vi "open SADI LV.vi"(10 "deviceNumber":i32, 11 "instance":i32) -> (3 "function return":u32)   [LabVIEW 2025, in "SADI_FW3.lvlib"]
doc: "SADI_API_Wrapper FT_STATUS openSADI_LV(int instance,int deviceNumber);"
uses:
  SADI_FW3.lvlib
  SADI_FW3.dll
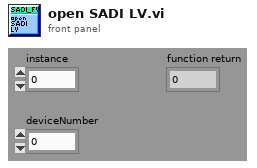
[diagram p1: front panel]
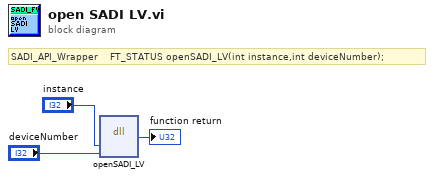
[diagram p0: block diagram]
diagram:
  # "SADI_API_Wrapper    FT_STATUS openSADI_LV(int instance,int deviceNumber);"
  n1 = dll-call lib="C:/Users/noaht/iCloudDrive/#1 School/Fall 2025/Controls Lab/LabView/EML4314c_FA25_framework_0/LVLib/SADI_FW3.*" fn="openSADI_LV"("instance"="instance", "deviceNumber"="deviceNumber") -> (→"function return":u32)  [unwired: 5 in, 2 out]
